vi "Open SpreadsheetDocument.vi"(7 "ooCalc":refnum<class "ooCalc.lvclass">, 8 "error in (no error)":errorcluster, 11 "filepath":path) -> (0 "error out":errorcluster, 3 "ooCalc out":refnum<class "ooCalc.lvclass">)   [LabVIEW 2009, in "ooCalc.lvclass"]
uses:
  ooCalc.lvclass
  C:/Projets/LAVAG/OpenOfficeRGT/AODL/DLLs/AODL.dll
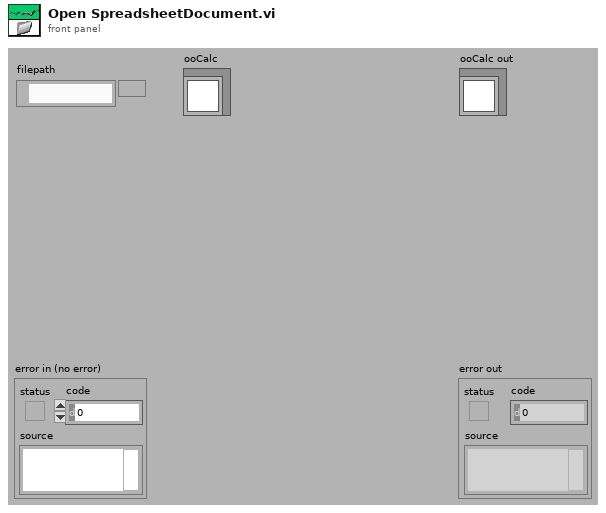
[diagram p1: front panel]
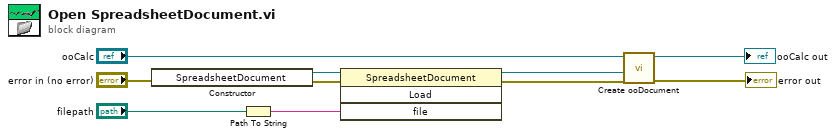
[diagram p0: block diagram]
diagram:
  n1 = constructor class="SpreadsheetDocument"(error in="error in (no error)") -> (reference out=w8:refnum<k24>, error out=w7:errorcluster)  [unwired: 2 in, 1 out]
  n2 = Path To String(path="filepath") -> (string=w9:string)
  n3 = invoke class="SpreadsheetDocument" method="Load"(reference=w8, error in=w7, "file"=w9) -> (reference out=w5:refnum<k24>, error out=w2:errorcluster)  [unwired: 1 in, 2 out]
  n4 = call-dynamic "Create ooDocument.vi"("error in (no error)"=w2, "Document"=w5, "ooDocument in"="ooCalc") -> ("error out"=→"error out":errorcluster, "ooDocument out"=→"ooCalc out":refnum<class "ooCalc.lvclass">)  [unwired: 7 in]
